vi "SimpleGyroLoop.vi"(8 "error in":errorcluster) -> ()   [LabVIEW 2014]
uses:
  <vilib>/Rock Robotics/WPI/Gyro/ADXRS453/WPI_Gyro_ADXRS453_Registers.ctl
  <vilib>/Platform/TimedLoop/XDataNode/timing_clust.ctl
  <vilib>/Platform/TimedLoop/XDataNode/nitl_modes.ctl
  <vilib>/Platform/TimedLoop/XDataNode/wakeup.ctl
  GyroGlobal.vi
  <vilib>/platform/TimedLoop/XDataNode/XDataNode.xnode
  <vilib>/Platform/TimedLoop/XDataNode/XDNodeRunTimeDep.lvlib
  <vilib>/ptbypt/NI_PtbyPt.lvlib
panel:
  out "mean":dbl format="%0.2f"
  in  "Calibrate":bool
  out "Angle":dbl
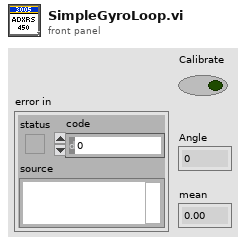
[diagram p1: front panel]
types:
  T1 = typedef "WPI_Gyro_ADXRS453_Registers.ctl" = u16
  T2 = typedef "WPI_SPIDevRef.ctl" = cluster{"DevStatus":errorcluster, "Handle":i32, "Controller":T3, "SPI Bus":T4}
  T3 = typedef "FPGA_TypedefDigitalModule.ctl" = enum16{"Controller 1"}
  T4 = typedef "spi_bus.ctl" = enum16{"SPI On-Board, CS0", "SPI On-Board, CS1", "SPI On-Board, CS2", "SPI On-Board, CS3", "SPI MXP", "Invalid"}
  T5 = typedef "XDNodeRunTimeDep.lvlib/timing_clust.ctl" = cluster{"Expected End [f-1]":u64, "Actual End [f-1]":u64, "Finished Late? [f-1]":bool, "Expected End [i-1]":u64, "Actual End [i-1]":u64, "Finished Late? [i-1]":bool, "Expected Start [i]":u64, "Actual Start [i]":u64, "Expected Start [f]":u64, "Actual Start [f]":u64, "Source Name":string, "Structure Name":string, "Period":i64, "Deadline":i64, "Offset":i64, "Start":i64, "Priority":i32, "Timeout":i32, "Mode":T6, "Wakeup Reason":T7, "Error":errorcluster, "Source Type":string, "Secondary Source Type":string, "Global End Time":u64, "Global Start Time":u64, "Frame Duration":u64, "Iteration Duration":u64, "Assigned CPU":i32, "I/O Scan Engine Mode":u32}
  T6 = typedef "XDNodeRunTimeDep.lvlib/nitl_modes.ctl" = enum32{"No Change", "Process missed periods, maintain original phase", "Discard missed periods, maintain original phase", "Process missed periods, ignore original phase", "Discard missed periods, ignore original phase"}
  T7 = typedef "XDNodeRunTimeDep.lvlib/wakeup.ctl" = enum32{"Normal", "Aborted", "Asynchronous wakeup", "Timing source error", "Timed loop error", "Timeout"}
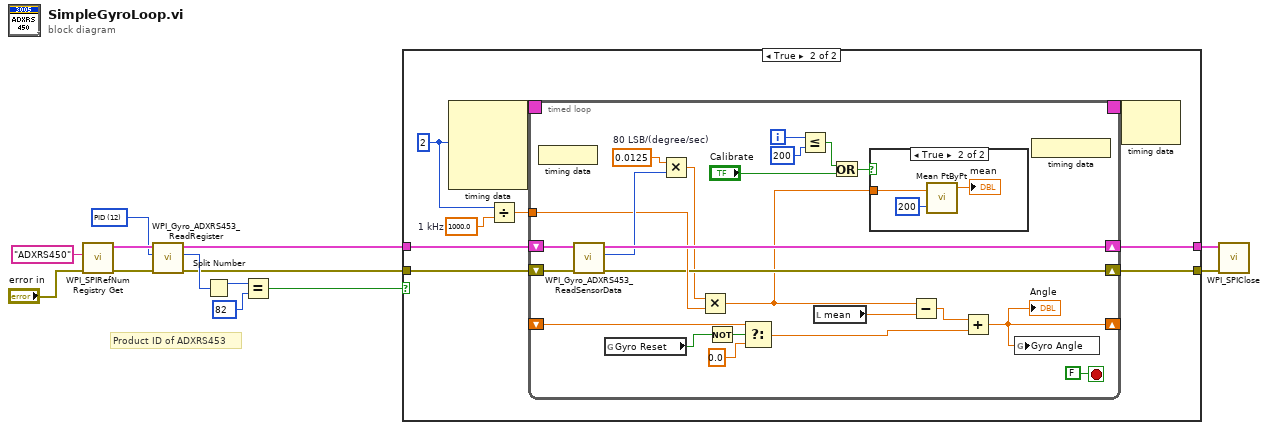
[diagram p0: block diagram]
diagram:
  w2 = T1 12 items=["Rate"=0, "Tem"=2, "LoCST"=4, "HiCST"=6, "Quad"=8, "Fault"=10, "PID"=12, "SN High"=14, "SN Low"=16]
  # "Product ID of ADXRS453"
  n1 = call <vilib>:"WPI_SPIRefNum Registry Get.vi"("error in (no error)"="error in", "refnum name"="ADXRS450") -> ("error out"=w12:errorcluster, "SPIDevRef"=w11:T2)  [unwired: 8 in]
  n2 = call <vilib>:"WPI_Gyro_ADXRS453_ReadRegister.vi"("error in (no error)"=w12, "ADXRS453 Register"=w2, "SPIDevRef in"=w11) -> ("error out"=w4:errorcluster, "Register Value"=w5:u16, "SPIDevRef out"=w3:T2)  [unwired: 6 in]
  n3 = Split Number(x=w5) -> (hi(x)=w6:u8)  [unwired: 1 out]
  n4 = Equal?(x=w6, y=u8 82) -> (x = y?=w10:bool)
  n5 = case shown="True" w10 {
    tunnel: w3 -> [w15 w22]
    tunnel: w4 -> [w14 w21]
    tunnel: [w14 w20] -> w8
    tunnel: [w15 w19] -> w9
    frame False {
    }
    frame True {
      w18 = 1000.0  # 1 kHz
      w16 = i64 2 ("Period")
      n6 = node-c288(w16) -> (w24:T5)  [unwired: 3 in]
      n7 = Divide(x=w16, y=w18) -> (x/y=w17:dbl)
      n8 = timed-loop {
        shift-right: [w45] -> w19
        shift-left: w22 -> [w47]
        shift-right: [w40] -> w20
        shift-left: w21 -> [w46]
        timing: w24 -> [_]
        timing-out: [_] -> w23
        shift-right: [w27] -> _
        shift-left: _ -> [w42]
        tunnel: w17 -> [w41]
        i -> [w30]
        stop <- FALSE stop-if-true
        w43 = 0.0125  # 80 LSB/(degree/sec)
        n9 = node-c288() -> ()  [unwired: 1 in]
        n10 = call <vilib>:"WPI_Gyro_ADXRS453_ReadSensorData.vi"("error in (no error)"=w46, "SPIDevRef in"=w47) -> ("error out"=w40:errorcluster, "Sensor Data (n-1)"=w44:i16, "SPIDevRef out"=w45:T2)  [unwired: 5 in, 2 out]
        n11 = global read "GyroGlobal.vi" "Gyro Reset"() -> (w26:bool)
        n12 = Multiply(x=w43, y=w44) -> (x*y=w37:dbl)
        n13 = Multiply(x=w37, y=w41) -> (x*y=w36:dbl)
        n14 = Not(x=w26) -> (.not. x?=w25:bool)
        n15 = Select(t=w42, s=w25, f=0.0 ("t")) -> (s? t:f=w34:dbl)
        n16 = Less Or Equal?(x=w30, y=200) -> (x <= y?=w28:bool)
        n17 = local read "mean"() -> (w32:dbl)
        n18 = Or(x=w28, y="Calibrate") -> (x .or. y?=w31:bool)
        n19 = case shown="True" w31 {
          tunnel: w36 -> [_ w49]
          frame False {
          }
          frame True {
            n20 = call <vilib>:"Mean PtByPt.vi"("x"=w49, "sample length"=200) -> ("mean"=→"mean":dbl)  [unwired: 2 in, 1 out]
          }
        }
        n21 = Subtract(x=w36, y=w32) -> (x-y=w39:dbl)
        n22 = Add(x=w39, y=w34) -> (x+y=w27:dbl)
        "Angle" <- w27
        n23 = global write "GyroGlobal.vi" "Gyro Angle"(w27) -> ()
        n24 = node-c288() -> ()  [unwired: 1 out]
      }
      n25 = node-c288(w23) -> ()  [unwired: 1 out]
    }
  }
  n26 = call <vilib>:"WPI_SPIClose.vi"("error in (no error)"=w8, "SPIDevRef"=w9) -> ()  [unwired: 9 in, 1 out]
